vi "ImageDistance.vi"(9 "Image 2":T1, 11 "Image 1":T1) -> (3 "Distance":dbl)   [LabVIEW 2015]
uses:
  <vilib>/vision/Image Controls.llb/IMAQ Image.ctl
  <vilib>/Analysis/baseanly.llb/Mean (DBL).vi
  <vilib>/Analysis/_algsub.llb/Real Vector Norm.vi
  <vilib>/Analysis/NI_AALBase.lvlib
  <vilib>/Analysis/NI_AALPro.lvlib
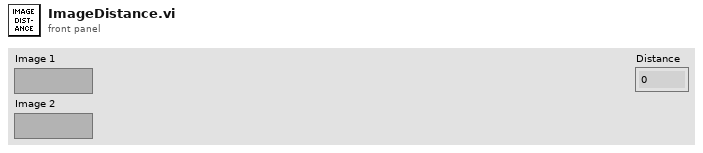
[diagram p1: front panel]
types:
  T1 = typedef "IMAQ Image.ctl" = refnum<image>
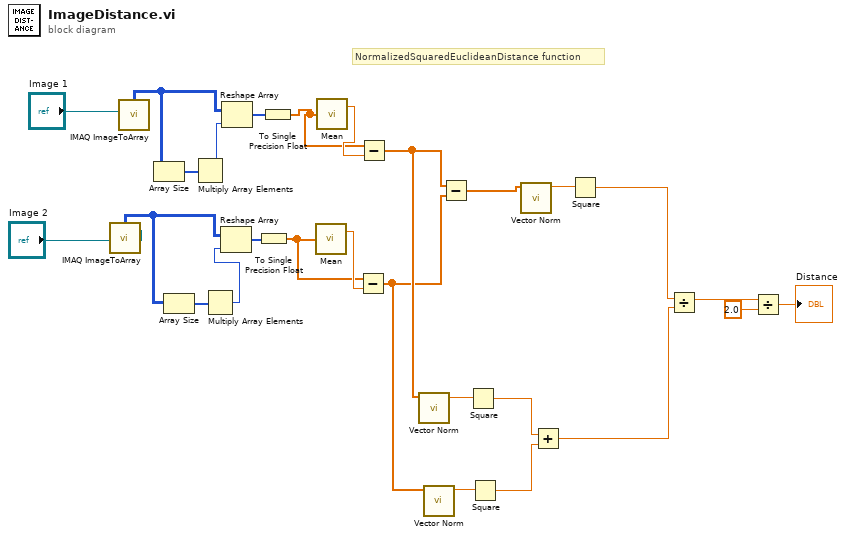
[diagram p0: block diagram]
diagram:
  # "NormalizedSquaredEuclideanDistance function"
  n1 = call "IMAQ ImageToArray"("Image"="Image 2") -> ("Image Pixels (U8)"=w6:u8[][])  [unwired: 3 in, 4 out]
  n2 = call "IMAQ ImageToArray"("Image"="Image 1") -> ("Image Pixels (U8)"=w2:u8[][])  [unwired: 3 in, 4 out]
  n3 = Array Size(array=w2) -> (size(s)=w3:i32[])
  n4 = Array Size(array=w6) -> (size(s)=w5:i32[])
  n5 = Multiply Array Elements(1:w3) -> (0:w1:i32)
  n6 = Multiply Array Elements(1:w5) -> (0:w4:i32)
  n7 = Reshape Array(w6, w4) -> (w10:u8[])
  n8 = Reshape Array(w2, w1) -> (w8:u8[])
  n9 = To Single Precision Float(number=w10) -> (single precision float=w9:sgl[])
  n10 = To Single Precision Float(number=w8) -> (single precision float=w7:sgl[])
  n11 = call-poly <vilib>:"Mean.vi"("X"=w9) -> ("mean"=w25:dbl)  [unwired: 1 out]
  n12 = call-poly <vilib>:"Mean.vi"("X"=w7) -> ("mean"=w24:dbl)  [unwired: 1 out]
  n13 = Subtract(x=w9, y=w25) -> (x-y=w20:dbl[])
  n14 = Subtract(x=w7, y=w24) -> (x-y=w21:dbl[])
  n15 = call-poly <vilib>:"Vector Norm.vi"("Input Vector"=w21) -> ("norm"=w18:dbl)  [unwired: 9 in, 1 out]
  n16 = call-poly <vilib>:"Vector Norm.vi"("Input Vector"=w20) -> ("norm"=w19:dbl)  [unwired: 9 in, 1 out]
  n17 = Subtract(x=w21, y=w20) -> (x-y=w23:dbl[])
  n18 = Square(x=w18) -> (x^2=w17:dbl)
  n19 = Square(x=w19) -> (x^2=w16:dbl)
  n20 = call-poly <vilib>:"Vector Norm.vi"("Input Vector"=w23) -> ("norm"=w22:dbl)  [unwired: 9 in, 1 out]
  n21 = Add(x=w17, y=w16) -> (x+y=w14:dbl)
  n22 = Square(x=w22) -> (x^2=w15:dbl)
  n23 = Divide(x=w15, y=w14) -> (x/y=w13:dbl)
  n24 = Divide(x=w13, y=2.0) -> (x/y=→"Distance":dbl)
